vi "Acquisition Complete.vi"(8 "error in (no error)":errorcluster, 11 "UserInterface in":refnum<class "UserInterface.lvclass">) -> (0 "error out":errorcluster, 3 "UserInterface out":refnum<class "UserInterface.lvclass">)   [LabVIEW 2022 SP3, in "UserInterface.lvlib" / "UserInterface.lvclass"]
uses:
  UserInterface.lvclass
  UserInterface.lvclass/UserInterface.ctl
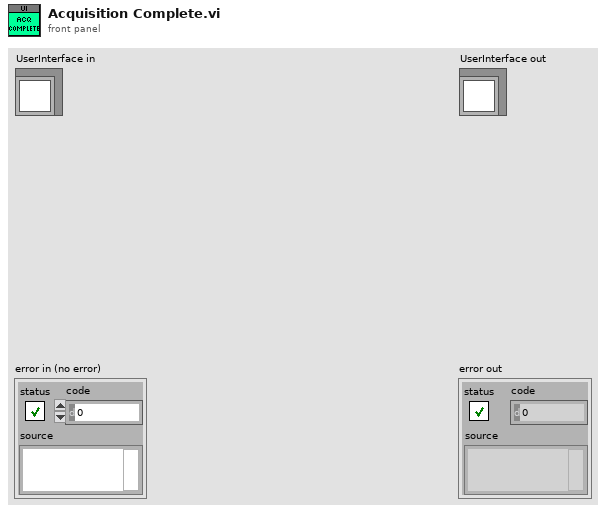
[diagram p1: front panel]
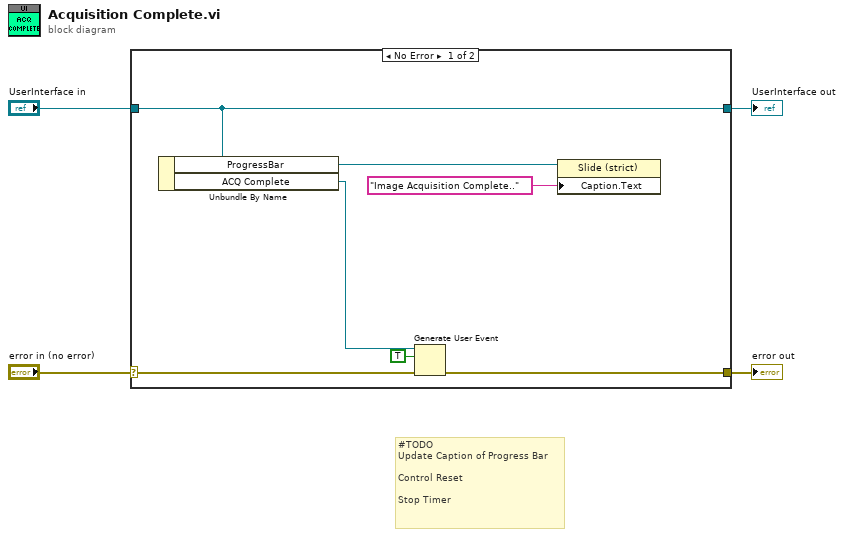
[diagram p0: block diagram]
diagram:
  # "#TODO \nUpdate Caption of Progress Bar\n\nControl Reset\n\nStop Timer"
  n1 = case shown="No Error" "error in (no error)" {
    selector: "error in (no error)" -> [w11 w13]
    tunnel: [w7 w13] -> w3
    tunnel: [w10 w12] -> w1
    tunnel: "UserInterface in" -> [w10 w12]
    frame No Error {
      n2 = Unbundle By Name(w10) -> ("ProgressBar"=w9:refnum<vi>, "ACQ Complete"=w6:refnum<user-event>)
      n3 = Generate User Event(user event=w6, event data cluster=TRUE ("event data"), error in=w11) -> (error out=w7:errorcluster)  [unwired: 1 in, 1 out]
      n4 = property class="Slide (strict)"(reference=w9, "Caption.Text"="Image Acquisition Complete..") -> ()  [unwired: 1 in, 2 out]
    }
    frame Error {
    }
  }
  "error out" <- w3
  "UserInterface out" <- w1
